vi "dfd_Calc Validated Order.vi"(7 "bank type":u16(ring) items=["2-band", "M-band Cosine-modulated PR"], 10 "bank counts":i32, 11 "order":i32) -> (1 "valid?":bool, 2 "validated order":i32, 3 "dup order":i32)   [LabVIEW 2017, in "NI_DigFilter_FilterBank.lvlib"]
uses:
  <vilib>/addons/Digital Filter Design/NI_DigFilter_FilterBank.lvlib
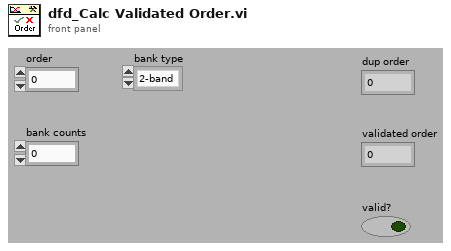
[diagram p1: front panel]
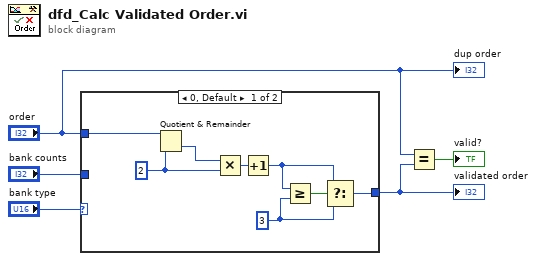
[diagram p0: block diagram]
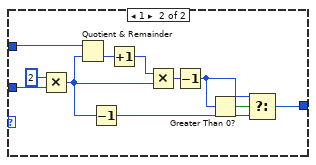
[diagram p2: hidden frame]
diagram:
  n1 = case shown="0, Default" "bank type" {
    tunnel: "order" -> [w6 w15]
    tunnel: [w7 w17] -> w2
    tunnel: "bank counts" -> [_ w21]
    frame 0, Default {
      w9 = 3
      w13 = 2
      n2 = Quotient & Remainder(x=w6, y=w13) -> (floor(x/y)=w12:i32)  [unwired: 1 out]
      n3 = Multiply(x=w12, y=w13) -> (x*y=w11:i32)
      n4 = Increment(x=w11) -> (x+1=w8:i32)
      n5 = Greater Or Equal?(x=w8, y=w9) -> (x >= y?=w10:bool)
      n6 = Select(t=w8, s=w10, f=w9) -> (s? t:f=w7:i32)
    }
    frame 1 {
      n7 = Multiply(x=2, y=w21) -> (x*y=w19:i32)
      n8 = Quotient & Remainder(x=w15, y=w19) -> (floor(x/y)=w24:i32)  [unwired: 1 out]
      n9 = Decrement(x=w19) -> (x-1=w18:i32)
      n10 = Increment(x=w24) -> (x+1=w14:i32)
      n11 = Multiply(x=w14, y=w19) -> (x*y=w23:i32)
      n12 = Decrement(x=w23) -> (x-1=w16:i32)
      n13 = Greater Than 0?(x=w16) -> (x > 0?=w20:bool)
      n14 = Select(t=w16, s=w20, f=w18) -> (s? t:f=w17:i32)
    }
  }
  "validated order" <- w2
  n15 = Equal?(x="order", y=w2) -> (x = y?=→"valid?":bool)
  "dup order" <- "order"
